vi "_PC_Toolbar_MSCmd_ActionEvent.vi"(6 "Interrupt Signal":refnum<vi>, 7 "exe param memory":T2, 8 "error in (no error)":errorcluster, 9 "Conn_Bool":refnum<data-value>, 10 "Cluster":T1, 11 "QMH In":refnum<class "QMH.lvclass">) -> ()   [LabVIEW 2018]
uses:
  PublicSubVI/Class/QMH/QMH.lvclass
  PublicSubVI/Ctl/RegistyFunc.ctl
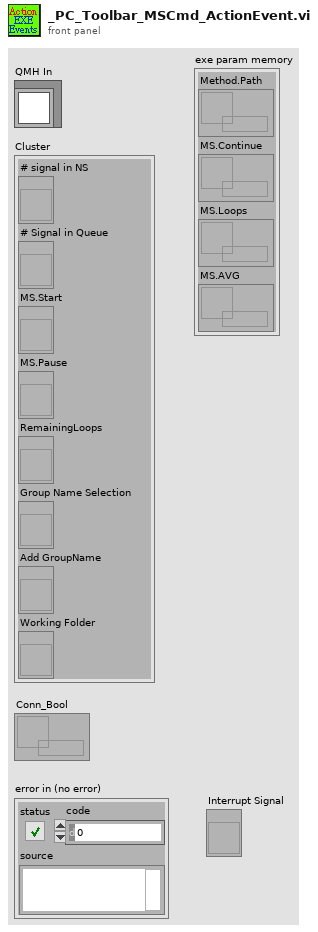
[diagram p1: front panel]
types:
  T1 = cluster{"# signal in NS":refnum<vi>, "# Signal in Queue":refnum<vi>, "MS.Start":refnum<vi>, "MS.Pause":refnum<vi>, "RemainingLoops":refnum<vi>, "Group Name Selection":refnum<vi>, "Add GroupName":refnum<vi>, "Working Folder":refnum<vi>}
  T2 = cluster{"Method.Path":refnum<data-value>, "MS.Continue":refnum<data-value>, "MS.Loops":refnum<data-value>, "MS.AVG":refnum<data-value>}
  T3 = cluster{"MassAnalExe?":refnum<k21>, "MassAnalPause":refnum<k21>, "MassAnalExe":refnum<k21>, "ExeTimes":refnum<k21>}
  T4 = enum8{"Enabled", "Disabled", "Disabled and Grayed Out"}
  T5 = enum16{"None", "Init", "Write", "Read", "PauseRead", "FinishCheck"}
  T6 = typedef "RegistyFunc.ctl" = enum16{"None", "FileAutoSave", "FileNoise", "FileSN", "ExeStatu", "WorkFolderPath", "MethodPath", "AVGItem", "LoopItem", "AutoRun", "BGColor", "LineColor", "LineWidth", "XGrid", "YGrid", "DeviceRefnum"}
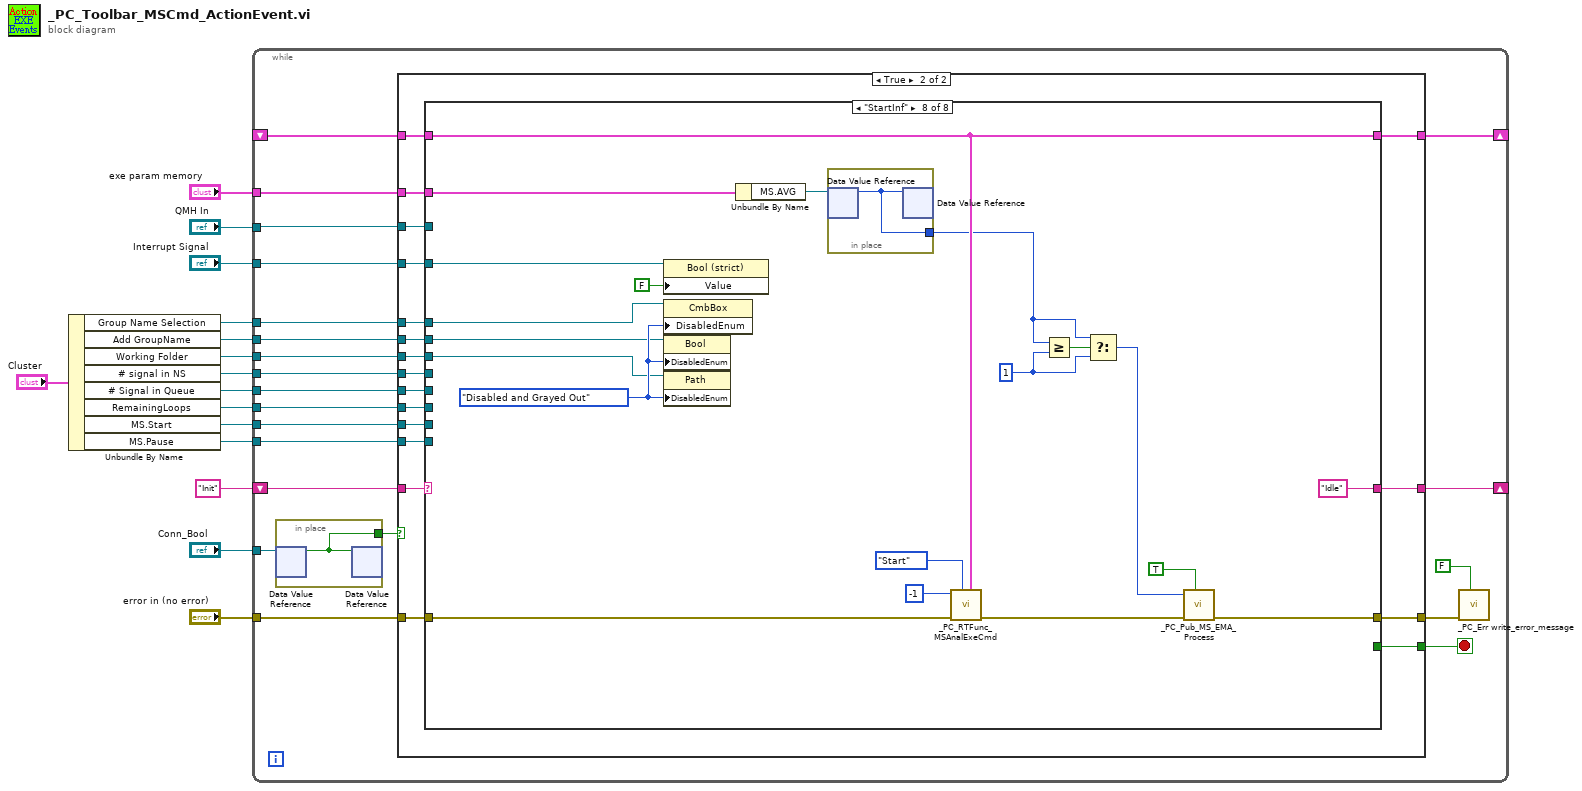
[diagram p0: block diagram]
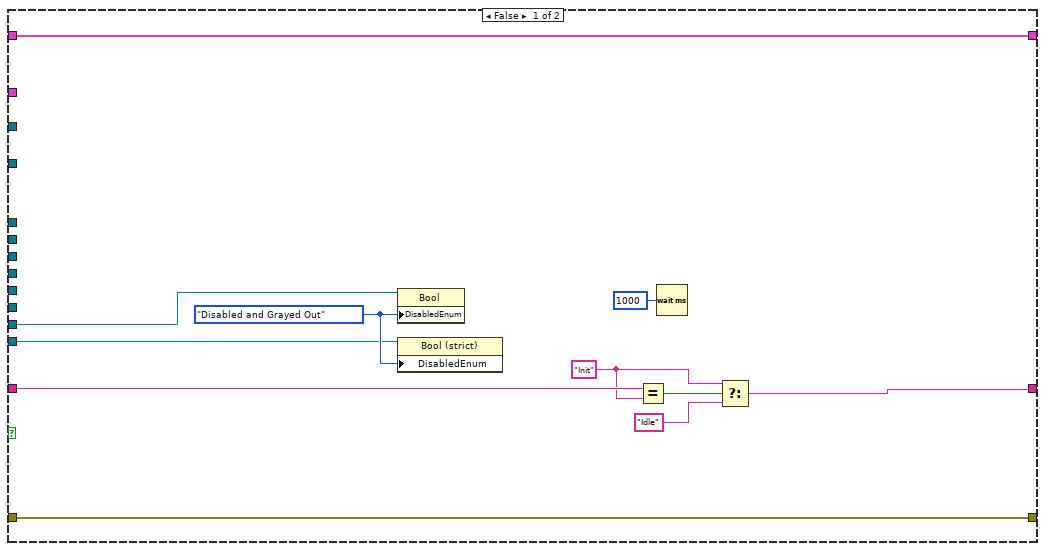
[diagram p2: hidden frame]
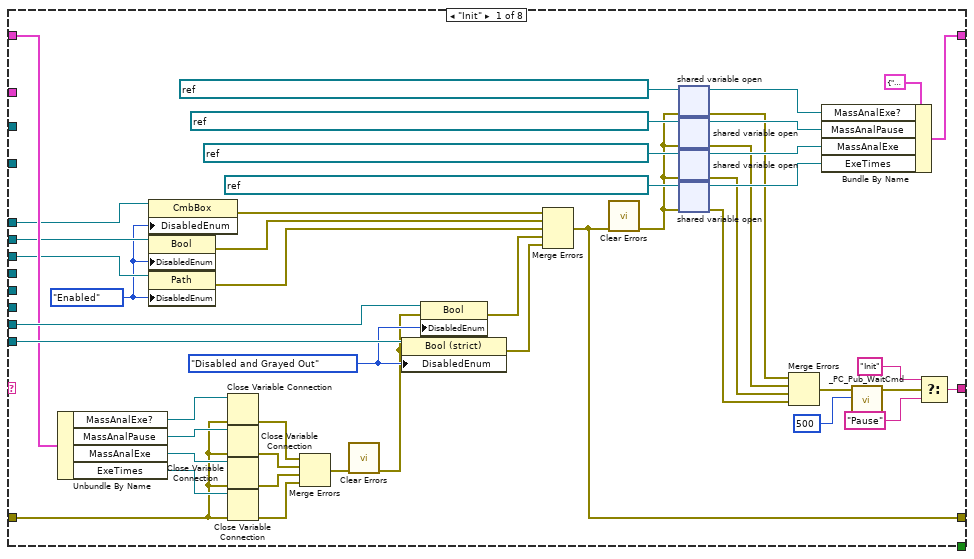
[diagram p3: hidden frame]
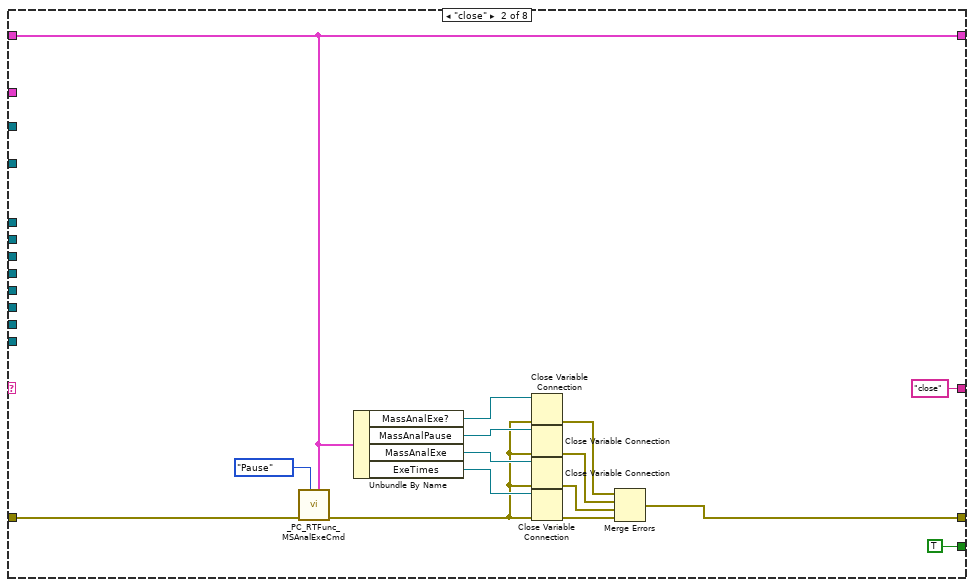
[diagram p4: hidden frame]
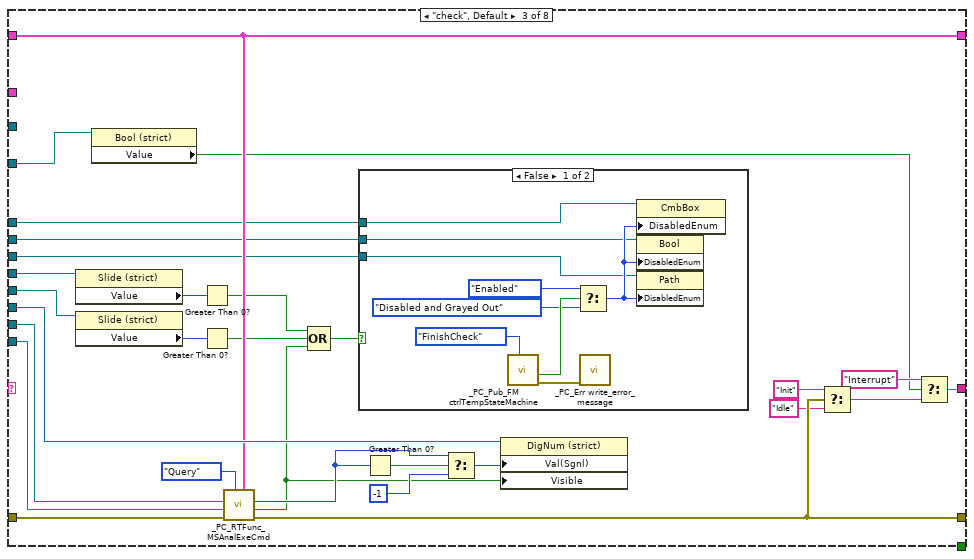
[diagram p5: hidden frame]
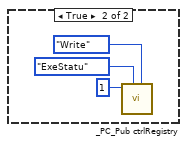
[diagram p6: hidden frame]
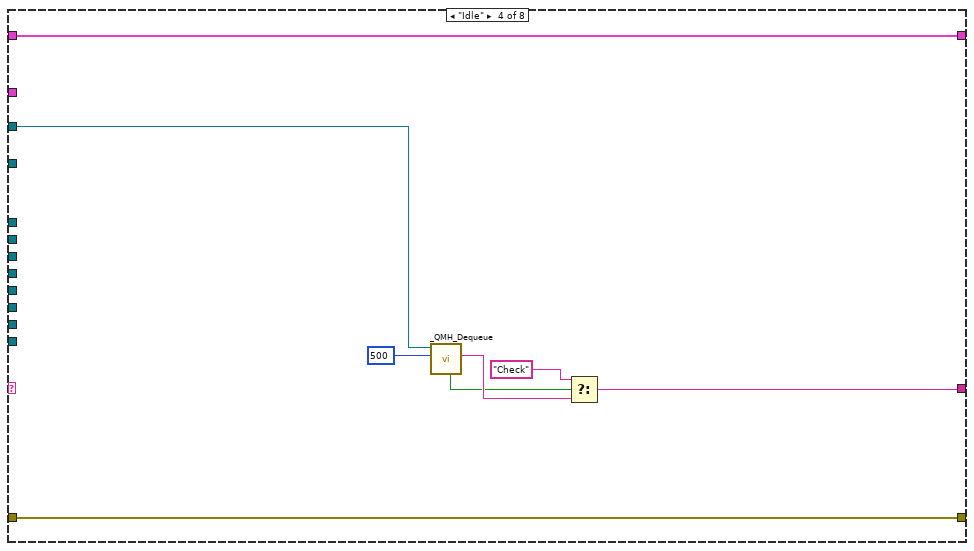
[diagram p7: hidden frame]
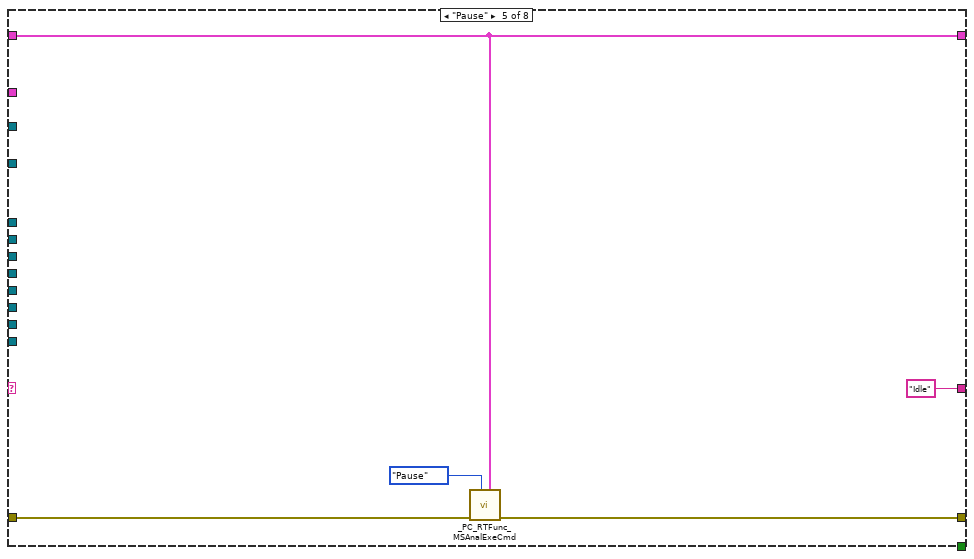
[diagram p8: hidden frame]
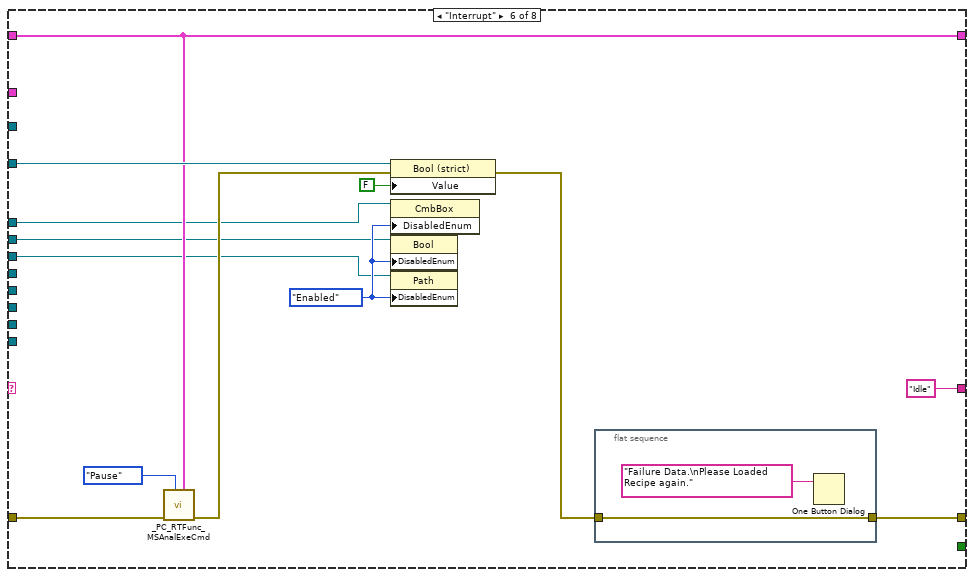
[diagram p9: hidden frame]
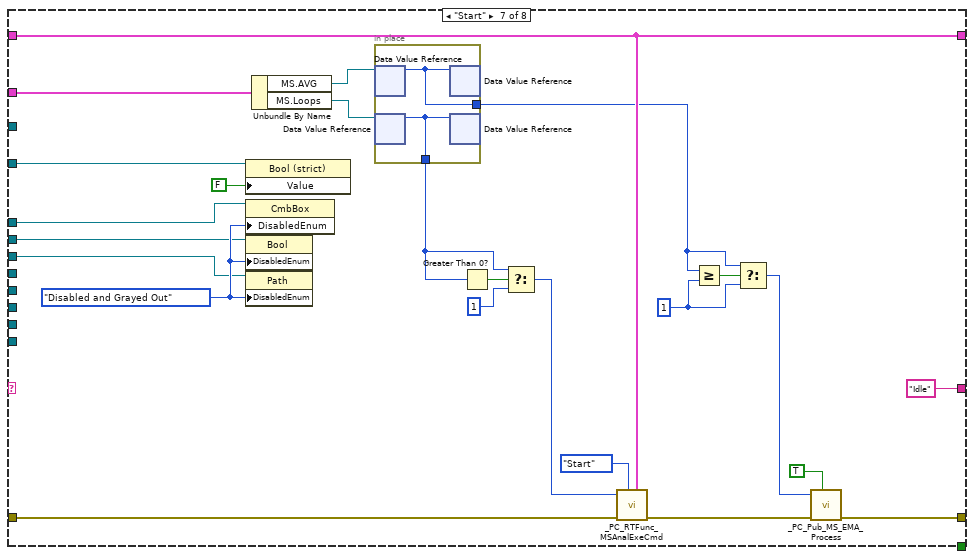
[diagram p10: hidden frame]
diagram:
  n1 = Unbundle By Name("Cluster") -> ("Group Name Selection"=w3:refnum<vi>, "Add GroupName"=w2:refnum<vi>, "Working Folder"=w1:refnum<vi>, "# signal in NS"=w13:refnum<vi>, "# Signal in Queue"=w12:refnum<vi>, "RemainingLoops"=w10:refnum<vi>, "MS.Start"=w8:refnum<vi>, "MS.Pause"=w7:refnum<vi>)
  n2 = while {
    tunnel: "QMH In" -> [w36]
    shift-right: [w28] -> _
    shift-left: "Init" ("Msg") -> [w35]
    tunnel: w8 -> [w34]
    tunnel: w7 -> [w33]
    tunnel: w13 -> [w32]
    tunnel: w12 -> [w31]
    tunnel: "error in (no error)" -> [w30]
    tunnel: "Conn_Bool" -> [w23]
    tunnel: "exe param memory" -> [w27]
    tunnel: w10 -> [w26]
    shift-right: [w25] -> _
    shift-left: _ -> [w24]
    tunnel: "Interrupt Signal" -> [w21]
    tunnel: w3 -> [w18]
    tunnel: w2 -> [w17]
    tunnel: w1 -> [w16]
    stop <- w19 stop-if-true
    n3 = in-place {
      in-place-border: [w243] -> w22
      n4 = in-place-dvr #1(w23) -> (w243:bool)  [unwired: 1 out]
      n5 = in-place-dvr #1(w243) -> ()  [unwired: 2 out]
    }
    n6 = case shown="True" w22 {
      tunnel: w36 -> [_ w65]
      tunnel: w35 -> [w44 w64]
      tunnel: w34 -> [w46 w63]
      tunnel: w33 -> [w45 w62]
      tunnel: w32 -> [_ w61]
      tunnel: w31 -> [_ w60]
      tunnel: w30 -> [w37 w59]
      tunnel: [w37 w58] -> w29
      tunnel: [w40 w57] -> w28
      tunnel: w27 -> [_ w56]
      tunnel: w26 -> [_ w55]
      tunnel: [w39 w54] -> w25
      tunnel: w24 -> [w39 w53]
      tunnel: w21 -> [_ w52]
      tunnel: [_ w51] -> w19
      tunnel: w18 -> [_ w50]
      tunnel: w17 -> [_ w49]
      tunnel: w16 -> [_ w48]
      frame False {
        w42 = "Init" ("y")
        w47 = T4."Disabled and Grayed Out" ("Disabled")
        n7 = property class="Bool"(reference=w46, "DisabledEnum"=w47) -> ()  [unwired: 1 in, 2 out]
        n8 = property class="Bool (strict)"(reference=w45, "DisabledEnum"=w47) -> ()  [unwired: 1 in, 2 out]
        n9 = Equal?(x=w44, y=w42) -> (x = y?=w43:bool)
        n10 = Wait (ms)(milliseconds to wait=u32 1000) -> ()  [unwired: 1 out]
        n11 = Select(t=w42, s=w43, f="Idle") -> (s? t:f=w40:string)
      }
      frame True {
        n12 = case shown="\"StartInf\"" w64 {
          tunnel: w65 -> [_ _ _ w175 _ _ _ _]
          tunnel: [w87 "close" ("Msg") w136 w174 "Idle" ("Msg") "Idle" ("Msg") "Idle" ("Msg") "Idle" ("Msg")] -> w57
          tunnel: w63 -> [w103 _ w148 _ _ _ _ _]
          tunnel: w62 -> [w102 _ w147 _ _ _ _ _]
          tunnel: w61 -> [_ _ w141 _ _ _ _ _]
          tunnel: w60 -> [_ _ w140 _ _ _ _ _]
          tunnel: w59 -> [w77 w113 w153 w168 w177 w189 w201 w239]
          tunnel: [w98 w117 w151 w168 w176 w186 w200 w227] -> w58
          tunnel: w56 -> [_ _ _ _ _ _ w212 w235]
          tunnel: w55 -> [_ _ w142 _ _ _ _ _]
          tunnel: [w99 w114 w139 w173 w178 w188 w208 w233] -> w54
          tunnel: w53 -> [w78 w114 w139 w173 w178 w188 w208 w233]
          tunnel: w52 -> [_ _ w134 _ _ w191 w207 w231]
          tunnel: [_ TRUE _ _ _ _ _ _] -> w51
          tunnel: w50 -> [w73 _ w129 _ _ w182 w198 w224]
          tunnel: w49 -> [w74 _ w128 _ _ w183 w197 w223]
          tunnel: w48 -> [w72 _ w127 _ _ w181 w196 w222]
          frame "Init" {
            w71 = T4."Enabled" ("Disabled")
            w101 = T4."Disabled and Grayed Out" ("Disabled")
            n13 = Unbundle By Name(w78) -> ("MassAnalExe?"=w86:refnum<k21>, "MassAnalPause"=w85:refnum<k21>, "MassAnalExe"=w84:refnum<k21>, "ExeTimes"=w83:refnum<k21>)
            n14 = property class="CmbBox"(reference=w73, "DisabledEnum"=w71) -> (error out=w70:errorcluster)  [unwired: 1 in, 1 out]
            n15 = property class="Bool"(reference=w74, "DisabledEnum"=w71) -> (error out=w69:errorcluster)  [unwired: 1 in, 1 out]
            n16 = property class="Path"(reference=w72, "DisabledEnum"=w71) -> (error out=w68:errorcluster)  [unwired: 1 in, 1 out]
            n17 = Close Variable Connection(8:w77, 11:w86) -> (0:w82:errorcluster)
            n18 = Close Variable Connection(8:w77, 11:w85) -> (0:w81:errorcluster)
            n19 = Close Variable Connection(8:w77, 11:w84) -> (0:w80:errorcluster)
            n20 = Close Variable Connection(8:w77, 11:w83) -> (0:w79:errorcluster)
            n21 = Merge Errors(w82, w81, w80, w79) -> (w76:errorcluster)
            n22 = call <vilib>:"Clear Errors.vi"("error in (no error)"=w76) -> ("error out"=w75:errorcluster)  [unwired: 5 in, 1 out]
            n23 = property class="Bool (strict)"(reference=w102, error in=w75, "DisabledEnum"=w101) -> (error out=w66:errorcluster)  [unwired: 1 out]
            n24 = property class="Bool"(reference=w103, error in=w75, "DisabledEnum"=w101) -> (error out=w67:errorcluster)  [unwired: 1 out]
            n25 = Merge Errors(w70, w69, w68, w67, w66) -> (w98:errorcluster)
            n26 = call <vilib>:"Clear Errors.vi"("error in (no error)"=w98) -> ("error out"=w100:errorcluster)  [unwired: 5 in, 1 out]
            n27 = shared-variable-open(refnum<k21> "ni.var.psp://NI-sbRIO/_RT_CtrlLoop_MassAnalysing_Variable/MassAnalExe%3F" ("shared variable refnum in"), w100) -> (w108:refnum<k21>, w96:errorcluster)
            n28 = shared-variable-open(refnum<k21> "ni.var.psp://NI-sbRIO/_RT_CtrlLoop_MassAnalysing_Variable/MassAnalPause" ("shared variable refnum in"), w100) -> (w109:refnum<k21>, w95:errorcluster)
            n29 = shared-variable-open(refnum<k21> "ni.var.psp://NI-sbRIO/_RT_CtrlLoop_MassAnalysing_Variable/MassAnalExe" ("shared variable refnum in"), w100) -> (w110:refnum<k21>, w94:errorcluster)
            n30 = shared-variable-open(refnum<k21> "ni.var.psp://NI-sbRIO/_RT_CtrlLoop_MassAnalysing_Variable/ExeTimes" ("shared variable refnum in"), w100) -> (w111:refnum<k21>, w93:errorcluster)
            n31 = Merge Errors(w96, w95, w94, w93) -> (w92:errorcluster)
            n32 = Bundle By Name(cluster=T3 {"MassAnalExe?"="", "MassAnalPause"="", "MassAnalExe"="", "ExeTimes"=""}, "MassAnalExe?"=w108, "MassAnalPause"=w109, "MassAnalExe"=w110, "ExeTimes"=w111) -> (w99:T3)
            n33 = call "_PC_Pub_WaitCmd.vi"("milliseconds to wait"=u32 500, "error in (no error)"=w92) -> ("error out"=w90:errorcluster)  [unwired: 9 in]
            n34 = Select(t="Init" ("Msg"), s=w90, f="Pause" ("Msg")) -> (s? t:f=w87:string)
          }
          frame "close" {
            n35 = call "_PC_RTFunc_MSAnalExeCmd.vi"("sv refnum"=w114, "Function"=enum16{"Query", "Start", "Pause"}."Pause", "error in (no error)"=w113) -> ("error out"=w112:errorcluster)  [unwired: 6 in, 2 out]
            n36 = Unbundle By Name(w114) -> ("MassAnalExe?"=w126:refnum<k21>, "MassAnalPause"=w125:refnum<k21>, "MassAnalExe"=w124:refnum<k21>, "ExeTimes"=w123:refnum<k21>)
            n37 = Close Variable Connection(8:w112, 11:w126) -> (0:w121:errorcluster)
            n38 = Close Variable Connection(8:w112, 11:w125) -> (0:w120:errorcluster)
            n39 = Close Variable Connection(8:w112, 11:w124) -> (0:w119:errorcluster)
            n40 = Close Variable Connection(8:w112, 11:w123) -> (0:w118:errorcluster)
            n41 = Merge Errors(w121, w120, w119, w118) -> (w117:errorcluster)
          }
          frame "check", Default {
            n42 = property class="Slide (strict)"(reference=w141) -> ("Value"=w152:u8)  [unwired: 1 in, 2 out]
            n43 = property class="Slide (strict)"(reference=w140) -> ("Value"=w154:u8)  [unwired: 1 in, 2 out]
            n44 = property class="Bool (strict)"(reference=w134) -> ("Value"=w133:bool)  [unwired: 1 in, 2 out]
            n45 = Greater Than 0?(x=w152) -> (x > 0?=w132:bool)
            n46 = Greater Than 0?(x=w154) -> (x > 0?=w131:bool)
            n47 = call "_PC_RTFunc_MSAnalExeCmd.vi"("sv refnum"=w139, "Function"=enum16{"Query", "Start", "Pause"}."Query", "error in (no error)"=w153, "MS.Pause"=w147, "MS.Start"=w148) -> ("error out"=w151:errorcluster, "MSAnalExe?"=w130:bool, "ExeTimes Out"=w144:i32)  [unwired: 4 in]
            n48 = Compound Arithmetic op=OR(w132, w131, w130) -> (w135:bool)
            n49 = case shown="False" w135 {
              tunnel: w129 -> [w156 _]
              tunnel: w128 -> [w157 _]
              tunnel: w127 -> [w158 _]
              frame False {
                n50 = call "_PC_Pub_FM ctrlTempStateMachine.vi"("function"=T5."FinishCheck") -> ("error out"=w160:errorcluster, "finish? (F)"=w163:bool)  [unwired: 8 in, 1 out]
                n51 = Select(t=T4."Enabled" ("Disabled"), s=w163, f=T4."Disabled and Grayed Out") -> (s? t:f=w159:T4)
                n52 = call "_PC_Err write_error_message.vi"("error in"=w160) -> ()  [unwired: 10 in, 1 out]
                n53 = property class="CmbBox"(reference=w156, "DisabledEnum"=w159) -> ()  [unwired: 1 in, 2 out]
                n54 = property class="Bool"(reference=w157, "DisabledEnum"=w159) -> ()  [unwired: 1 in, 2 out]
                n55 = property class="Path"(reference=w158, "DisabledEnum"=w159) -> ()  [unwired: 1 in, 2 out]
              }
              frame True {
                n56 = call "_PC_Pub ctrlRegistry.vi"("type"=enum16{"None", "Write", "Read"}."Write", "function"=RegistyFunc."ExeStatu", "write value"=u32 1) -> ()  [unwired: 5 in, 4 out]
              }
            }
            n57 = Greater Than 0?(x=w144) -> (x > 0?=w146:bool)
            n58 = Select(t=w144, s=w146, f=-1) -> (s? t:f=w143:i32)
            n59 = property class="DigNum (strict)"(reference=w142, "Val(Sgnl)"=w143, "Visible"=w130) -> ()  [unwired: 1 in, 2 out]
            n60 = Select(t="Init" ("Msg"), s=w151, f="Idle" ("Msg")) -> (s? t:f=w137:string)
            n61 = Select(t="Interrupt", s=w133, f=w137) -> (s? t:f=w136:string)
          }
          frame "Idle" {
            n62 = call "_QMH_Dequeue.vi"("timeout in ms (-1)"=500, "QMH in"=w175) -> ("Msg"=w171:string, "timed out?"=w169:bool)  [unwired: 4 in, 4 out]
            n63 = Select(t="Check", s=w169, f=w171) -> (s? t:f=w174:string)
          }
          frame "Pause" {
            n64 = call "_PC_RTFunc_MSAnalExeCmd.vi"("sv refnum"=w178, "Function"=enum16{"Query", "Start", "Pause"}."Pause", "error in (no error)"=w177) -> ("error out"=w176:errorcluster)  [unwired: 6 in, 2 out]
          }
          frame "Interrupt" {
            w184 = T4."Enabled" ("Disabled")
            n65 = call "_PC_RTFunc_MSAnalExeCmd.vi"("sv refnum"=w188, "Function"=enum16{"Query", "Start", "Pause"}."Pause", "error in (no error)"=w189) -> ("error out"=w187:errorcluster)  [unwired: 6 in, 2 out]
            n66 = property class="Bool (strict)"(reference=w191, error in=w187, "Value"=FALSE) -> (error out=w185:errorcluster)  [unwired: 1 out]
            n67 = property class="CmbBox"(reference=w182, "DisabledEnum"=w184) -> ()  [unwired: 1 in, 2 out]
            n68 = property class="Bool"(reference=w183, "DisabledEnum"=w184) -> ()  [unwired: 1 in, 2 out]
            n69 = property class="Path"(reference=w181, "DisabledEnum"=w184) -> ()  [unwired: 1 in, 2 out]
            n70 = flat-sequence {
              tunnel: w185 -> [w195]
              tunnel: [w195] -> w186
              frame #0 {
                n71 = One Button Dialog(message="Failure Data.\nPlease Loaded Recipe again.") -> ()  [unwired: 1 in, 1 out]
              }
            }
          }
          frame "Start" {
            w199 = T4."Disabled and Grayed Out" ("Disabled")
            w202 = 1 ("f")
            n72 = property class="Bool (strict)"(reference=w207, "Value"=FALSE) -> ()  [unwired: 1 in, 2 out]
            n73 = property class="CmbBox"(reference=w198, "DisabledEnum"=w199) -> ()  [unwired: 1 in, 2 out]
            n74 = property class="Bool"(reference=w197, "DisabledEnum"=w199) -> ()  [unwired: 1 in, 2 out]
            n75 = property class="Path"(reference=w196, "DisabledEnum"=w199) -> ()  [unwired: 1 in, 2 out]
            n76 = Unbundle By Name(w212) -> ("MS.AVG"=w209:refnum<data-value>, "MS.Loops"=w211:refnum<data-value>)
            n77 = in-place {
              in-place-border: [w221] -> w210
              in-place-border: [w220] -> w203
              n78 = in-place-dvr #2(w209) -> (w220:u8)  [unwired: 1 out]
              n79 = in-place-dvr #3(w211) -> (w221:i32)  [unwired: 1 out]
              n80 = in-place-dvr #2(w220) -> ()  [unwired: 2 out]
              n81 = in-place-dvr #3(w221) -> ()  [unwired: 2 out]
            }
            n82 = Greater Than 0?(x=w210) -> (x > 0?=w218:bool)
            n83 = Select(t=w210, s=w218, f=1) -> (s? t:f=w216:i32)
            n84 = call "_PC_RTFunc_MSAnalExeCmd.vi"("sv refnum"=w208, "Function"=enum16{"Query", "Start", "Pause"}."Start", "error in (no error)"=w201, "Loops in"=w216) -> ("error out"=w214:errorcluster)  [unwired: 5 in, 2 out]
            n85 = Greater Or Equal?(x=w203, y=w202) -> (x >= y?=w205:bool)
            n86 = Select(t=w203, s=w205, f=w202) -> (s? t:f=w204:i32)
            n87 = call "_PC_Pub_MS_EMA_Process.vi"("Init? ( F )"=TRUE ("Init?"), "error in (no error)"=w214, "AVGValue"=w204) -> ("error out"=w200:errorcluster)  [unwired: 6 in, 2 out]
          }
          frame "StartInf" {
            w225 = T4."Disabled and Grayed Out" ("Disabled")
            w229 = 1 ("f")
            n88 = property class="Bool (strict)"(reference=w231, "Value"=FALSE) -> ()  [unwired: 1 in, 2 out]
            n89 = property class="CmbBox"(reference=w224, "DisabledEnum"=w225) -> ()  [unwired: 1 in, 2 out]
            n90 = property class="Bool"(reference=w223, "DisabledEnum"=w225) -> ()  [unwired: 1 in, 2 out]
            n91 = property class="Path"(reference=w222, "DisabledEnum"=w225) -> ()  [unwired: 1 in, 2 out]
            n92 = Unbundle By Name(w235) -> ("MS.AVG"=w234:refnum<data-value>)
            n93 = in-place {
              in-place-border: [w242] -> w226
              n94 = in-place-dvr #4(w234) -> (w242:u8)  [unwired: 1 out]
              n95 = in-place-dvr #4(w242) -> ()  [unwired: 2 out]
            }
            n96 = call "_PC_RTFunc_MSAnalExeCmd.vi"("sv refnum"=w233, "Function"=enum16{"Query", "Start", "Pause"}."Start", "error in (no error)"=w239, "Loops in"=-1) -> ("error out"=w237:errorcluster)  [unwired: 5 in, 2 out]
            n97 = Greater Or Equal?(x=w226, y=w229) -> (x >= y?=w230:bool)
            n98 = Select(t=w226, s=w230, f=w229) -> (s? t:f=w228:i32)
            n99 = call "_PC_Pub_MS_EMA_Process.vi"("Init? ( F )"=TRUE ("Init?"), "error in (no error)"=w237, "AVGValue"=w228) -> ("error out"=w227:errorcluster)  [unwired: 6 in, 2 out]
          }
        }
      }
    }
    n100 = call "_PC_Err write_error_message.vi"("show msg( T )"=FALSE, "error in"=w29) -> ()  [unwired: 9 in, 1 out]
  }
